vi "format_AnMiTC_data.vi"(8 "index":i32, 10 "value_array":dbl[](array[numeric]), 11 "time":timestamp) -> (1 "value":dbl, 3 "waveform_array":waveform(dbl)[](array[waveform])=[{"t0"=timestamp(0 s since 1904-01-01), "dt"=1.0, "Y"=[]}, {"t0"=timestamp(3732035173.078092 s since 1904-01-01), "dt"=1.0, "Y"=[302.8589782714844], "attributes"=variant("NI_ChannelName"=variant(string "T1"))}])   [LabVIEW 2019]
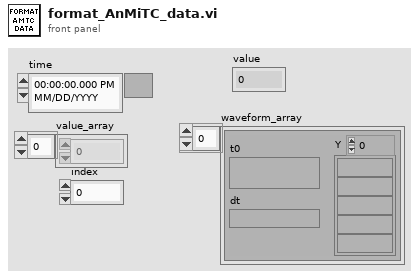
[diagram p1: front panel]
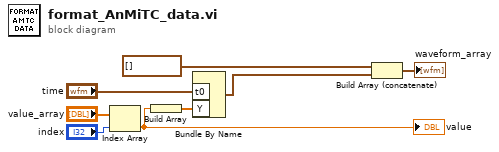
[diagram p0: block diagram]
diagram:
  n1 = Index Array(array="value_array", index="index") -> (element=w3:dbl)
  "value" <- w3
  n2 = Build Array(w3) -> (w7:dbl[])
  n3 = Bundle By Name("t0"="time", "Y"=w7) -> (w6:waveform(dbl))  [unwired: 1 in]
  n4 = Build Array (concatenate)(waveform(dbl)[] [], w6) -> (→"waveform_array":waveform(dbl)[])
